vi "UMLEditor_ColorsDialog.vi"(5 "error in (no error)":errorcluster) -> (19 "error out":errorcluster)   [LabVIEW 2016]
doc: "Helpinstructions."
uses:
  <resource>/Framework/Providers/Open_GDS/UML/UMLEditor/UMLEditor_StoredColors.ctl
  <resource>/Framework/Providers/Open_GDS/ClassProviders/Common/CommonVIs/CommonVIs_ColorMemoryAction.ctl
panel:
  in  "State Background Color":u32(colorbox)
  in  "Class Background Color (for <<TYPE>> Stereotype)":u32(colorbox)
  in  "Class Background Color (for <<Application/VI>> Stereotype)":u32(colorbox)
  in  "Class Background Color (with class/vi path, but no class found)":u32(colorbox)
  in  "Class Background Color":u32(colorbox)
  in  "Classes":string(tree) caption="These classes could be converted to use a relative path"
  in  "Ok":bool
  in  "Cancel":bool
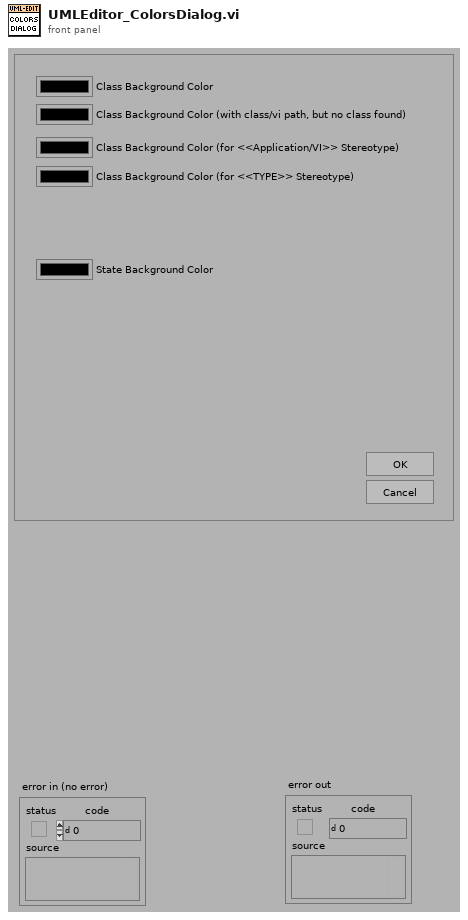
[diagram p1: front panel]
types:
  T1 = typedef "UMLEditor_StoredColors.ctl" = enum16{"ClassBackgroudColor", "ClassBackgroudColorWithClassPath", "ClassBackgroudColorForApplicationVIStereotype", "ClassBackgroudColorForTypeStereotype", "StateBackgroudColor"}
  T2 = typedef "CommonVIs_ColorMemoryAction.ctl" = enum16{"Get Color", "Set Color", "Delete Color", "Clear All Colors"}
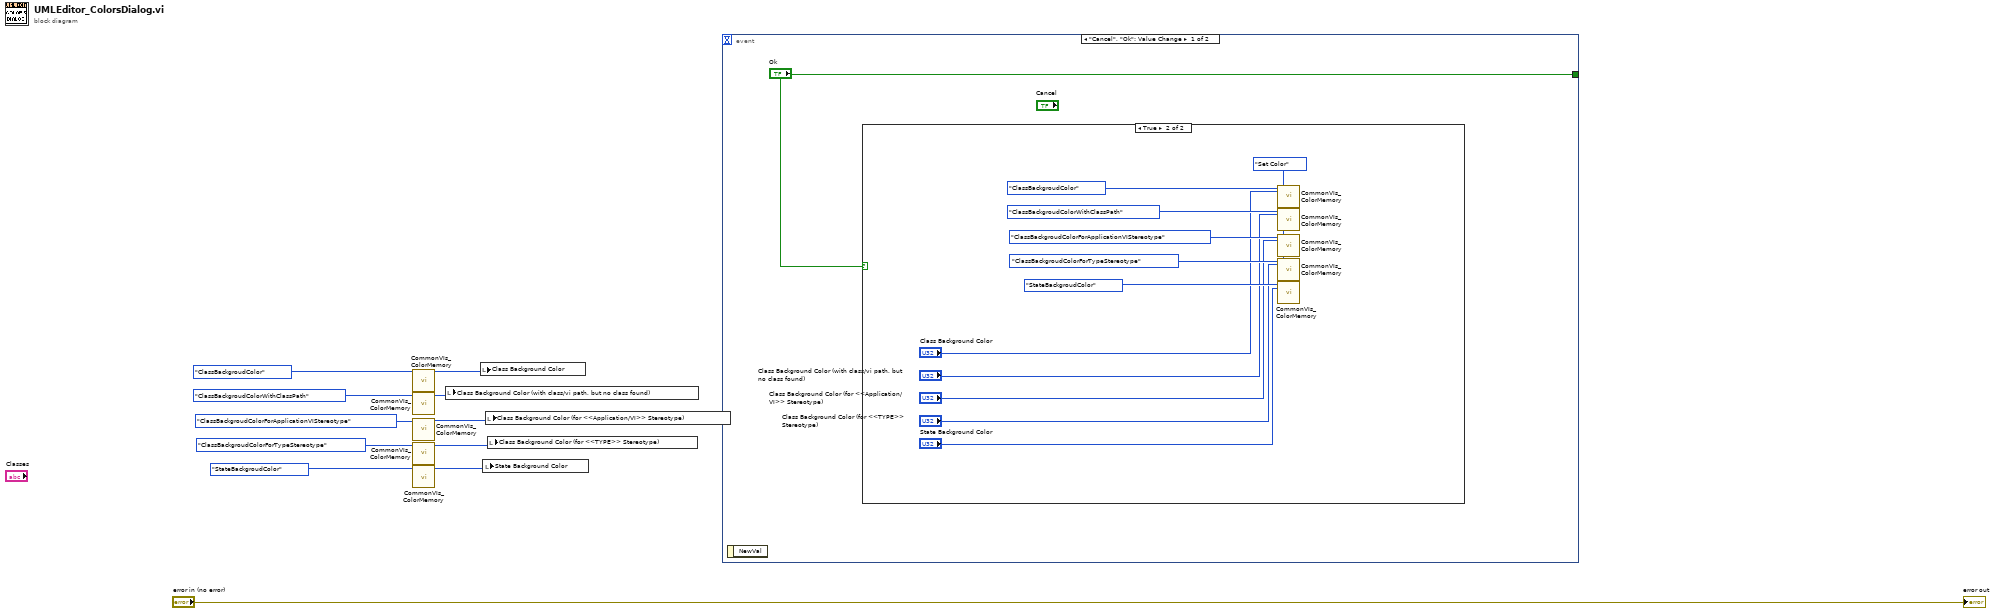
[diagram p0: block diagram]
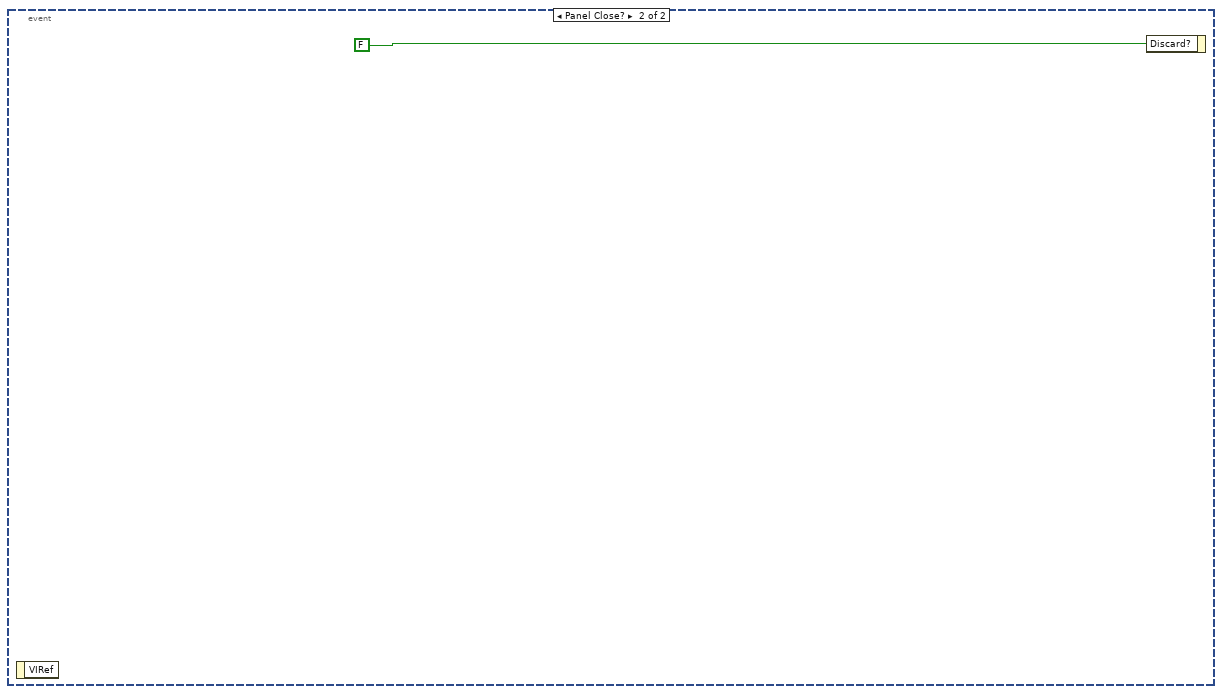
[diagram p3: hidden frame]
diagram:
  n1 = call <resource>:"CommonVIs_ColorMemory.vi"("ColorName"=UMLEditor_StoredColors."ClassBackgroudColor" ("UMLPathes")) -> ("Color Out"=w9:u32)  [unwired: 3 in, 15 out]
  n2 = call <resource>:"CommonVIs_ColorMemory.vi"("ColorName"=UMLEditor_StoredColors."ClassBackgroudColorWithClassPath" ("UMLPathes")) -> ("Color Out"=w8:u32)  [unwired: 3 in, 15 out]
  n3 = call <resource>:"CommonVIs_ColorMemory.vi"("ColorName"=UMLEditor_StoredColors."ClassBackgroudColorForApplicationVIStereotype" ("UMLPathes")) -> ("Color Out"=w7:u32)  [unwired: 3 in, 15 out]
  n4 = call <resource>:"CommonVIs_ColorMemory.vi"("ColorName"=UMLEditor_StoredColors."ClassBackgroudColorForTypeStereotype" ("UMLPathes")) -> ("Color Out"=w6:u32)  [unwired: 3 in, 15 out]
  n5 = call <resource>:"CommonVIs_ColorMemory.vi"("ColorName"=UMLEditor_StoredColors."StateBackgroudColor" ("UMLPathes")) -> ("Color Out"=w2:u32)  [unwired: 3 in, 15 out]
  n6 = local write "Class Background Color (with class/vi path, but no class found)"(w8) -> ()
  n7 = local write "Class Background Color"(w9) -> ()
  n8 = local write "State Background Color"(w2) -> ()
  n9 = local write "Class Background Color (for <<Application/VI>> Stereotype)"(w7) -> ()
  n10 = local write "Class Background Color (for <<TYPE>> Stereotype)"(w6) -> ()
  n11 = event shown="[0] \"Cancel\", \"Ok\": Value Change" {
    selector: _ -> [_ _]
    dyn-events: _ -> [_ _]
    timeout: _ -> [_ _]
    tunnel: ["Ok" _] -> _
    event "Cancel", "Ok": Value Change {
      n12 = event-data() -> ()  [unwired: 2 out]
      n13 = case shown="True" "Ok" {
        frame False {
        }
        frame True {
          w15 = CommonVIs_ColorMemoryAction."Set Color" ("Method (Get Color)")
          n14 = call <resource>:"CommonVIs_ColorMemory.vi"("ColorName"=UMLEditor_StoredColors."ClassBackgroudColor" ("UMLPathes"), "Color In"="Class Background Color", "Method (Get Color)"=w15) -> ()  [unwired: 1 in, 16 out]
          n15 = call <resource>:"CommonVIs_ColorMemory.vi"("ColorName"=UMLEditor_StoredColors."ClassBackgroudColorWithClassPath" ("UMLPathes"), "Color In"="Class Background Color (with class/vi path, but no class found)", "Method (Get Color)"=w15) -> ()  [unwired: 1 in, 16 out]
          n16 = call <resource>:"CommonVIs_ColorMemory.vi"("ColorName"=UMLEditor_StoredColors."ClassBackgroudColorForApplicationVIStereotype" ("UMLPathes"), "Color In"="Class Background Color (for <<Application/VI>> Stereotype)", "Method (Get Color)"=w15) -> ()  [unwired: 1 in, 16 out]
          n17 = call <resource>:"CommonVIs_ColorMemory.vi"("ColorName"=UMLEditor_StoredColors."ClassBackgroudColorForTypeStereotype" ("UMLPathes"), "Color In"="Class Background Color (for <<TYPE>> Stereotype)", "Method (Get Color)"=w15) -> ()  [unwired: 1 in, 16 out]
          n18 = call <resource>:"CommonVIs_ColorMemory.vi"("ColorName"=UMLEditor_StoredColors."StateBackgroudColor" ("UMLPathes"), "Color In"="State Background Color", "Method (Get Color)"=w15) -> ()  [unwired: 1 in, 16 out]
        }
      }
    }
    event Panel Close? {
      n19 = event-data() -> ()  [unwired: 2 out]
      n20 = event-data("Discard?"=FALSE) -> ()  [unwired: 1 in, 1 out]
    }
  }
  "error out" <- "error in (no error)"
